vi "Ketihley_read_data.vi"(0 "refnum":refnum<file>) -> ()   [LabVIEW 2019]
uses:
  Global/Global Variables/Data_Display_global.vi
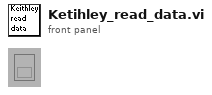
[diagram p1: front panel]
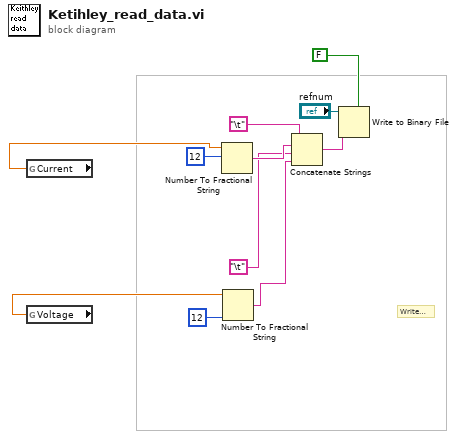
[diagram p0: block diagram]
diagram:
  # "Write File"
  n1 = global read "Data_Display_global.vi" "Current"() -> (w4:dbl)
  n2 = global read "Data_Display_global.vi" "Voltage"() -> (w3:dbl)
  n3 = Number To Fractional String(number=w4, precision (6)=i16 12) -> (F-format string=w8:string)  [unwired: 2 in]
  n4 = Number To Fractional String(number=w3, precision (6)=i16 12) -> (F-format string=w1:string)  [unwired: 2 in]
  n5 = Concatenate Strings("\t", w8, "\t", w1) -> (w10:string)
  n6 = Write to Binary File ("Write File")(file (use dialog)="refnum", data=w10, 5:FALSE ("prepend array or string size? (T)")) -> ()  [unwired: 3 in, 3 out]
